vi "Write Test Group Manager.vi"(8 "error in (no error)":errorcluster, 10 "Test Group Manager":refnum<data-value>, 11 "QPA Measurement in":refnum<class "QPA Measurement.lvclass">) -> (0 "error out":errorcluster, 3 "QPA Measurement out":refnum<class "QPA Measurement.lvclass">)   [LabVIEW 2016, in "QPA Measurement.lvlib" / "QPA Measurement.lvclass"]
uses:
  QPA Measurement.lvclass
  Plugins/Test Group Manager.lvlibp/Test Group Manager.lvclass
  QPA Measurement.lvclass/QPA Measurement.ctl
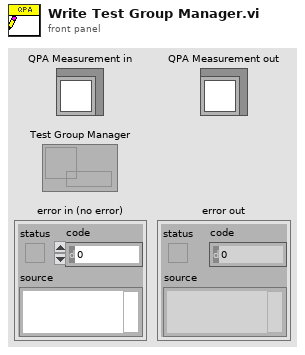
[diagram p1: front panel]
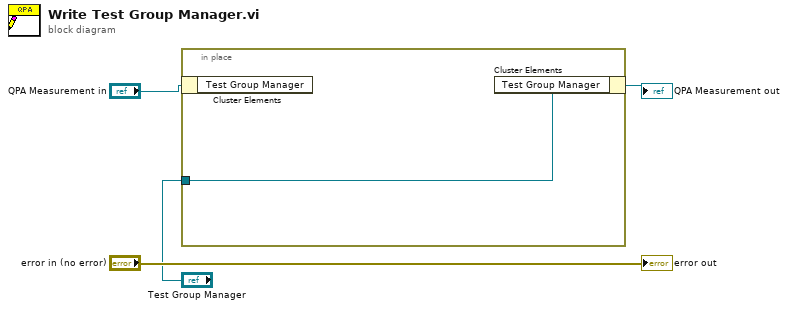
[diagram p0: block diagram]
diagram:
  n1 = in-place {
    in-place-border: "Test Group Manager" -> [w5]
    n2 = in-place-cluster #1("QPA Measurement in") -> ()  [unwired: 1 out]
    n3 = in-place-cluster #1("Test Group Manager"=w5) -> (→"QPA Measurement out":refnum<class "QPA Measurement.lvclass">)
  }
  "error out" <- "error in (no error)"
